vi "getChildArray.vi"(8 "error in (no error)":errorcluster, 11 "NativeXML in":refnum<class "NativeXML.lvclass">) -> (0 "error out":errorcluster, 2 "childArray":refnum<class "NativeXML.lvclass">[](array[class]), 3 "NativeXML out":refnum<class "NativeXML.lvclass">)   [LabVIEW 2011, in "Tools.lvlib" / "xml.lvlib" / "NativeXML.lvclass"]
uses:
  NativeXML.lvclass
  NativeXML.lvclass/NativeXML.ctl
  <vilib>/xml/NI_XML.lvlib
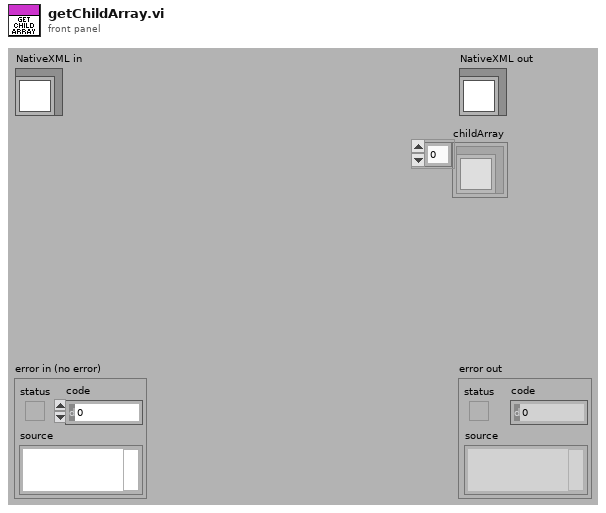
[diagram p1: front panel]
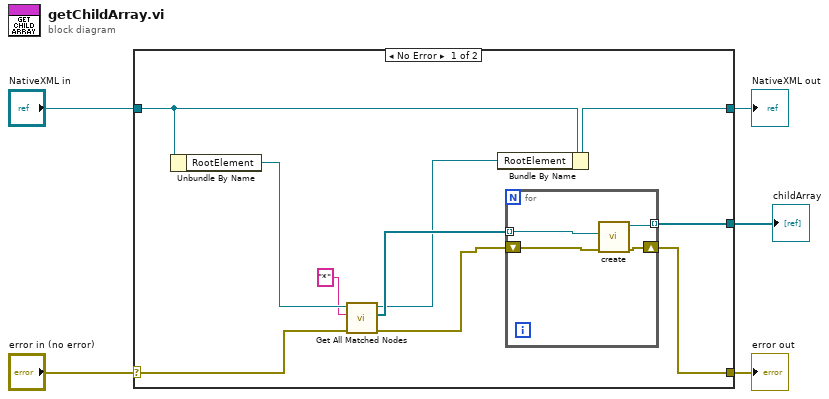
[diagram p0: block diagram]
diagram:
  n1 = case shown="No Error" "error in (no error)" {
    selector: "error in (no error)" -> [w10 w21]
    tunnel: [w13 w21] -> w4
    tunnel: [w14 w20] -> w2
    tunnel: "NativeXML in" -> [w15 w20]
    tunnel: [w12 _] -> w1
    frame No Error {
      n2 = Unbundle By Name(w15) -> ("RootElement"=w11:refnum<k20>)
      n3 = call <vilib>:"Get All Matched Nodes.vi"("error in (no error)"=w10, "XPath expression"="*", "node in"=w11) -> ("error out"=w8:errorcluster, "node result array"=w7:refnum<k20>[], "node out"=w6:refnum<k20>)  [unwired: 6 in]
      n4 = Bundle By Name(cluster=w15, "RootElement"=w6) -> (w14:refnum<class "NativeXML.lvclass">)
      n5 = for {
        tunnel: w7 -> [w17] mode=indexing
        shift-right: [w19] -> w13
        shift-left: w8 -> [w18]
        tunnel: [w16] -> w12 mode=indexing
        n6 = call "create.vi"("error in (no error)"=w18, "RootElement"=w17) -> ("error out"=w19:errorcluster, "NativeXML out"=w16:refnum<class "NativeXML.lvclass">)  [unwired: 8 in]
      }
    }
    frame Error {
    }
  }
  "error out" <- w4
  "NativeXML out" <- w2
  "childArray" <- w1
